vi "CascadedRC.vi"(8 "init/cont (init:F)":bool=TRUE, 9 "N. stages":u32=2, 10 "IIR Filter in":T1, 11 "X":cdb[](array[numeric])=[1.0+1.0i, 1.0+1.0i, 1.0+1.0i, 1.0+1.0i, 1.0+1.0i, 1.0+1.0i, 1.0+1.0i, 1.0+1.0i, 1.0+1.0i, 1.0+1.0i, 1.0+1.0i, 1.0+1.0i, 1.0+1.0i, 1.0+1.0i, 1.0+1.0i, 1.0+1.0i, 1.0+1.0i, 1.0+1.0i, 1.0+1.0i, 1.0+1.0i, 1.0+1.0i, 1.0+1.0i, 1.0+1.0i, 1.0+1.0i, 1.0+1.0i, 1.0+1.0i, 1.0+1.0i, 1.0+1.0i, 1.0+1.0i, 1.0+1.0i, 1.0+1.0i, 1.0+1.0i, 1.0+1.0i, 1.0+1.0i, 1.0+1.0i, 1.0+1.0i, 1.0+1.0i, 1.0+1.0i, 1.0+1.0i, 1.0+1.0i, 1.0+1.0i, 1.0+1.0i, 1.0+1.0i, 1.0+1.0i, 1.0+1.0i, 1.0+1.0i, 1.0+1.0i, 1.0+1.0i, 1.0+1.0i, 1.0+1.0i, 1.0+1.0i, 1.0+1.0i, 1.0+1.0i, 1.0+1.0i, 1.0+1.0i, 1.0+1.0i, 1.0+1.0i, 1.0+1.0i, 1.0+1.0i, 1.0+1.0i, 1.0+1.0i, 1.0+1.0i, 1.0+1.0i, 1.0+1.0i, 1.0+1.0i, 1.0+1.0i, 1.0+1.0i, 1.0+1.0i, 1.0+1.0i, 1.0+1.0i, 1.0+1.0i, 1.0+1.0i, 1.0+1.0i, 1.0+1.0i, 1.0+1.0i, 1.0+1.0i, 1.0+1.0i, 1.0+1.0i, 1.0+1.0i, 1.0+1.0i, 1.0+1.0i, 1.0+1.0i, 1.0+1.0i, 1.0+1.0i, 1.0+1.0i, 1.0+1.0i, 1.0+1.0i, 1.0+1.0i, 1.0+1.0i, 1.0+1.0i, 1.0+1.0i, 1.0+1.0i, 1.0+1.0i, 1.0+1.0i, 1.0+1.0i, 1.0+1.0i, 1.0+1.0i, 1.0+1.0i, 1.0+1.0i, 1.0+1.0i, 1.0+1.0i, 1.0+1.0i, 1.0+1.0i, 1.0+1.0i, 1.0+1.0i, 1.0+1.0i, 1.0+1.0i, 1.0+1.0i, 1.0+1.0i, 1.0+1.0i, 1.0+1.0i, 1.0+1.0i, 1.0+1.0i, 1.0+1.0i, 1.0+1.0i, 1.0+1.0i, 1.0+1.0i, 1.0+1.0i, 1.0+1.0i, 1.0+1.0i, 1.0+1.0i, 1.0+1.0i, 1.0+1.0i, 1.0+1.0i, 1.0+1.0i, 1.0+1.0i, 1.0+1.0i, 1.0+1.0i, 1.0+1.0i, 1.0+1.0i, 1.0+1.0i, 1.0+1.0i, 1.0+1.0i, 1.0+1.0i, 1.0+1.0i, 1.0+1.0i, 1.0+1.0i, 1.0+1.0i, 1.0+1.0i, 1.0+1.0i, 1.0+1.0i, 1.0+1.0i, 1.0+1.0i, 1.0+1.0i, 1.0+1.0i, 1.0+1.0i, 1.0+1.0i, 1.0+1.0i, 1.0+1.0i, 1.0+1.0i, 1.0+1.0i, 1.0+1.0i, 1.0+1.0i, 1.0+1.0i, 1.0+1.0i, 1.0+1.0i, 1.0+1.0i, 1.0+1.0i, 1.0+1.0i, 1.0+1.0i, 1.0+1.0i, 1.0+1.0i, 1.0+1.0i, 1.0+1.0i, 1.0+1.0i, 1.0+1.0i, 1.0+1.0i, 1.0+1.0i, 1.0+1.0i, 1.0+1.0i, 1.0+1.0i, 1.0+1.0i, 1.0+1.0i, 1.0+1.0i, 1.0+1.0i, 1.0+1.0i, 1.0+1.0i, 1.0+1.0i, 1.0+1.0i, 1.0+1.0i, 1.0+1.0i, 1.0+1.0i, 1.0+1.0i, 1.0+1.0i, 1.0+1.0i, 1.0+1.0i, 1.0+1.0i, 1.0+1.0i, 1.0+1.0i, 1.0+1.0i, 1.0+1.0i, 1.0+1.0i, 1.0+1.0i, 1.0+1.0i, 1.0+1.0i, 1.0+1.0i, 1.0+1.0i, 1.0+1.0i, 1.0+1.0i, 1.0+1.0i, 1.0+1.0i, 1.0+1.0i, 1.0+1.0i, 1.0+1.0i, 1.0+1.0i, 1.0+1.0i, 1.0+1.0i, 1.0+1.0i, 1.0+1.0i, 1.0+1.0i, 1.0+1.0i, 1.0+1.0i, 1.0+1.0i, 1.0+1.0i, 1.0+1.0i, 1.0+1.0i, 1.0+1.0i, 1.0+1.0i, 1.0+1.0i, 1.0+1.0i, 1.0+1.0i, 1.0+1.0i, 1.0+1.0i, 1.0+1.0i, 1.0+1.0i, 1.0+1.0i, 1.0+1.0i, 1.0+1.0i, 1.0+1.0i, 1.0+1.0i, 1.0+1.0i, 1.0+1.0i, 1.0+1.0i, 1.0+1.0i, 1.0+1.0i, 1.0+1.0i, 1.0+1.0i, 1.0+1.0i, 1.0+1.0i, 1.0+1.0i, 1.0+1.0i, 1.0+1.0i, 1.0+1.0i, 1.0+1.0i, 1.0+1.0i, 1.0+1.0i, 1.0+1.0i, 1.0+1.0i, 1.0+1.0i, 1.0+1.0i, 1.0+1.0i, 1.0+1.0i, 1.0+1.0i, 1.0+1.0i, 1.0+1.0i, 1.0+1.0i, 1.0+1.0i, 1.0+1.0i, 1.0+1.0i, 1.0+1.0i, 1.0+1.0i, 1.0+1.0i, 1.0+1.0i, 1.0+1.0i, 1.0+1.0i, 1.0+1.0i, 1.0+1.0i, 1.0+1.0i, 1.0+1.0i, 1.0+1.0i, 1.0+1.0i, 1.0+1.0i, 1.0+1.0i, 1.0+1.0i, 1.0+1.0i, 1.0+1.0i, 1.0+1.0i, 1.0+1.0i, 1.0+1.0i, 1.0+1.0i, 1.0+1.0i, 1.0+1.0i, 1.0+1.0i, 1.0+1.0i, 1.0+1.0i, 1.0+1.0i, 1.0+1.0i, 1.0+1.0i, 1.0+1.0i, 1.0+1.0i, 1.0+1.0i, 1.0+1.0i, 1.0+1.0i, 1.0+1.0i, 1.0+1.0i, 1.0+1.0i, 1.0+1.0i, 1.0+1.0i, 1.0+1.0i, 1.0+1.0i, 1.0+1.0i, 1.0+1.0i, 1.0+1.0i, 1.0+1.0i, 1.0+1.0i, 1.0+1.0i, 1.0+1.0i, 1.0+1.0i, 1.0+1.0i, 1.0+1.0i, 1.0+1.0i, 1.0+1.0i, 1.0+1.0i, 1.0+1.0i, 1.0+1.0i, 1.0+1.0i, 1.0+1.0i, 1.0+1.0i, 1.0+1.0i, 1.0+1.0i, 1.0+1.0i, 1.0+1.0i, 1.0+1.0i, 1.0+1.0i, 1.0+1.0i, 1.0+1.0i, 1.0+1.0i, 1.0+1.0i, 1.0+1.0i, 1.0+1.0i, 1.0+1.0i, 1.0+1.0i, 1.0+1.0i, 1.0+1.0i, 1.0+1.0i, 1.0+1.0i, 1.0+1.0i, 1.0+1.0i, 1.0+1.0i, 1.0+1.0i, 1.0+1.0i, 1.0+1.0i, 1.0+1.0i, 1.0+1.0i, 1.0+1.0i, 1.0+1.0i, 1.0+1.0i, 1.0+1.0i, 1.0+1.0i, 1.0+1.0i, 1.0+1.0i, 1.0+1.0i, 1.0+1.0i, 1.0+1.0i, 1.0+1.0i, 1.0+1.0i, 1.0+1.0i, 1.0+1.0i, 1.0+1.0i, 1.0+1.0i, 1.0+1.0i, 1.0+1.0i, 1.0+1.0i, 1.0+1.0i, 1.0+1.0i, 1.0+1.0i, 1.0+1.0i, 1.0+1.0i, 1.0+1.0i, 1.0+1.0i, 1.0+1.0i, 1.0+1.0i, 1.0+1.0i, 1.0+1.0i, 1.0+1.0i, 1.0+1.0i, 1.0+1.0i, 1.0+1.0i, 1.0+1.0i, 1.0+1.0i, 1.0+1.0i, 1.0+1.0i, 1.0+1.0i, 1.0+1.0i, 1.0+1.0i, 1.0+1.0i, 1.0+1.0i, 1.0+1.0i, 1.0+1.0i, 1.0+1.0i, 1.0+1.0i, 1.0+1.0i, 1.0+1.0i, 1.0+1.0i, 1.0+1.0i, 1.0+1.0i, 1.0+1.0i, 1.0+1.0i, 1.0+1.0i, 1.0+1.0i, 1.0+1.0i, 1.0+1.0i, 1.0+1.0i, 1.0+1.0i, 1.0+1.0i, 1.0+1.0i, 1.0+1.0i, 1.0+1.0i, 1.0+1.0i, 1.0+1.0i, 1.0+1.0i, 1.0+1.0i, 1.0+1.0i, 1.0+1.0i, 1.0+1.0i, 1.0+1.0i, 1.0+1.0i, 1.0+1.0i, 1.0+1.0i, 1.0+1.0i, 1.0+1.0i, 1.0+1.0i, 1.0+1.0i, 1.0+1.0i, 1.0+1.0i, 1.0+1.0i, 1.0+1.0i, 1.0+1.0i, 1.0+1.0i, 1.0+1.0i, 1.0+1.0i, 1.0+1.0i, 1.0+1.0i, 1.0+1.0i, 1.0+1.0i, 1.0+1.0i, 1.0+1.0i, 1.0+1.0i, 1.0+1.0i, 1.0+1.0i, 1.0+1.0i, 1.0+1.0i, 1.0+1.0i, 1.0+1.0i, 1.0+1.0i, 1.0+1.0i, 1.0+1.0i, 1.0+1.0i, 1.0+1.0i, 1.0+1.0i, 1.0+1.0i, 1.0+1.0i, 1.0+1.0i, 1.0+1.0i, 1.0+1.0i, 1.0+1.0i, 1.0+1.0i, 1.0+1.0i, 1.0+1.0i, 1.0+1.0i, 1.0+1.0i, 1.0+1.0i, 1.0+1.0i, 1.0+1.0i, 1.0+1.0i, 1.0+1.0i, 1.0+1.0i, 1.0+1.0i, 1.0+1.0i, 1.0+1.0i, 1.0+1.0i, 1.0+1.0i, 1.0+1.0i, 1.0+1.0i, 1.0+1.0i, 1.0+1.0i, 1.0+1.0i, 1.0+1.0i, 1.0+1.0i, 1.0+1.0i, 1.0+1.0i, 1.0+1.0i, 1.0+1.0i, 1.0+1.0i, 1.0+1.0i, 1.0+1.0i, 1.0+1.0i, 1.0+1.0i, 1.0+1.0i, 1.0+1.0i, 1.0+1.0i, 1.0+1.0i, 1.0+1.0i, 1.0+1.0i]) -> (3 "Filtered X":cdb[](array[numeric]))   [LabVIEW 2019]
uses:
  <vilib>/Analysis/baseanly.llb/IIR Cascade Filter (CDB).vi
  <vilib>/Analysis/NI_AALBase.lvlib
panel:
  out "Waveform Graph":dbl[][](graph)
  out "All stages":cdb[][](array[numeric])
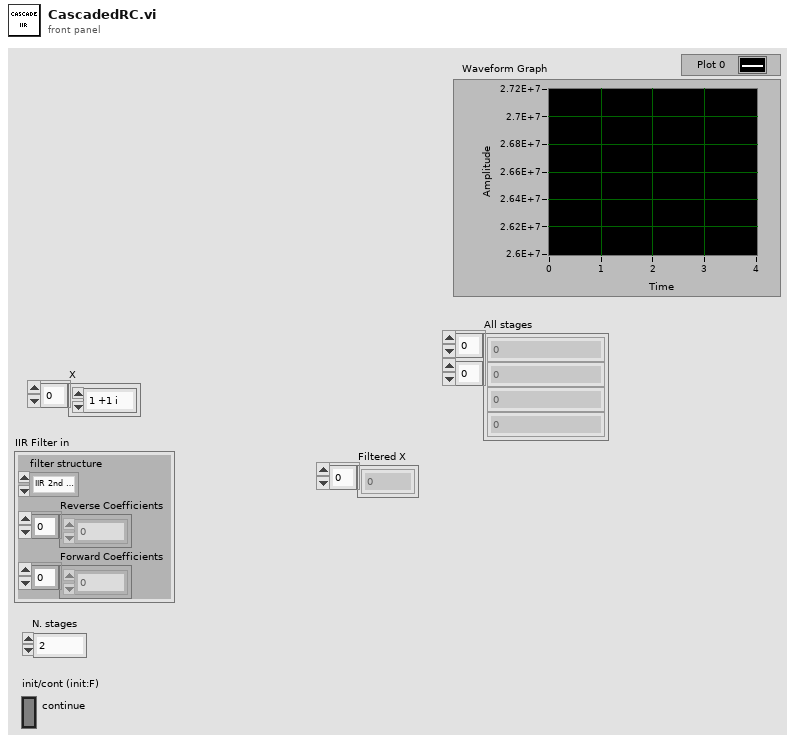
[diagram p1: front panel]
types:
  T1 = cluster{"filter structure":enum32{"IIR 2nd Order", "IIR 4th Order"}, "Reverse Coefficients":dbl[], "Forward Coefficients":dbl[]}
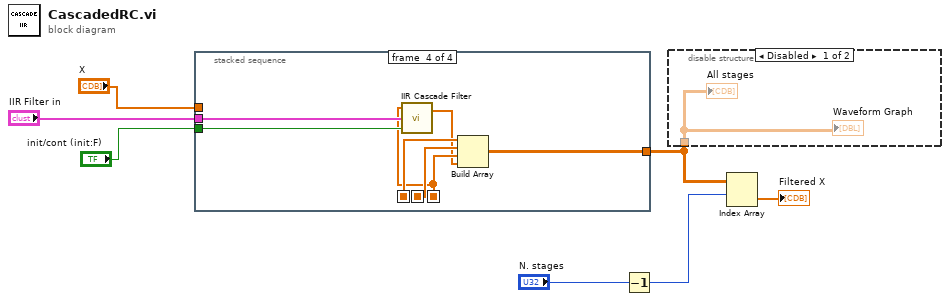
[diagram p0: block diagram]
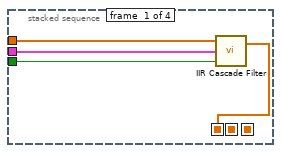
[diagram p3: hidden frame]
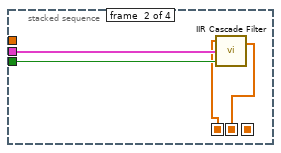
[diagram p4: hidden frame]
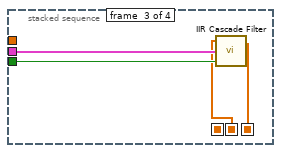
[diagram p5: hidden frame]
diagram:
  n1 = stacked-sequence {
    seq-local: [w8 _ _ _] -> [_ w12 _ w24]
    seq-local: [_ w13 _ _] -> [_ _ w16 w23]
    seq-local: [_ _ w17 _] -> [_ _ _ w22]
    tunnel: "X" -> [w11 _ _ _]
    tunnel: "IIR Filter in" -> [w10 w15 w19 w26]
    tunnel: "init/cont (init:F)" -> [w9 w14 w18 w25]
    tunnel: [_ _ _ w20] -> w1
    frame #0 {
      n2 = call-poly <vilib>:"IIR Cascade Filter.vi"("init/cont (init:F)"=w9, "IIR Filter Cluster"=w10, "X"=w11) -> ("Filtered X"=w8:cdb[])  [unwired: 1 out]
    }
    frame #1 {
      n3 = call-poly <vilib>:"IIR Cascade Filter.vi"("init/cont (init:F)"=w14, "IIR Filter Cluster"=w15, "X"=w12) -> ("Filtered X"=w13:cdb[])  [unwired: 1 out]
    }
    frame #2 {
      n4 = call-poly <vilib>:"IIR Cascade Filter.vi"("init/cont (init:F)"=w18, "IIR Filter Cluster"=w19, "X"=w16) -> ("Filtered X"=w17:cdb[])  [unwired: 1 out]
    }
    frame #3 {
      n5 = call-poly <vilib>:"IIR Cascade Filter.vi"("init/cont (init:F)"=w25, "IIR Filter Cluster"=w26, "X"=w22) -> ("Filtered X"=w21:cdb[])  [unwired: 1 out]
      n6 = Build Array(w24, w23, w22, w21) -> (w20:cdb[][])
    }
  }
  n7 = Decrement(x="N. stages") -> (x-1=w3:u32)
  n8 = disable-structure shown="Disabled" {
    disable-tunnel: w1 -> [w27 _]
    frame Disabled {
      "All stages" <- w27
      "Waveform Graph" <- w27
    }
    frame Enabled {
    }
  }
  n9 = Index Array(array=w1, index (row)=w3) -> (element=→"Filtered X":cdb[])  [unwired: 1 in]
